vi "oopAPI_TX (SAP)_2.vi"() -> ()   [LabVIEW 2020]
uses:
  src/_polimorphicInstances/control/Fdx Start (Tx).vi
  src/AIM664LV.lvlib
  src/_polimorphicInstances/session/Fdx Close Session (Port).vi
  src/_polimorphicInstances/session/Fdx Create Session (Tx-UDP Port-Oriented).vi
  src/helpers/EthFrameManagement/EthFrameManagement.lvlib
  src/bsp/AFDX_Transmit/Fdx Create Tx VL.vi
  src/_polimorphicInstances/udpPort/Fdx Create UDP Port (TX-SAP).vi
  src/_polimorphicInstances/control/Fdx Stop (Tx).vi
  src/_controls/comm_config_vl_tx.ctl
  src/_controls/sap_config_tx.ctl
  src/_controls/comm_computedMAC-IP.ctl
panel:
  out "Duplicated":bool
  out "Array":T1[](array[typedef]) {"MACsrc" format="%.0x"}
  in  "SapPort Config":T2[](array[typedef])=[{"partitionID"=1, "SubVlId"=1, "UdpSrcPort"=1, "UdpNumBufMessages"=0, "UdpMaxMessageSize"=1000}]
  in  "VL Config":T3={"VlId"=60, "NumOfSubVl"=1, "rate mS (128)"=128.0, "domainID"=1, "sideID"=1, "locationID"=1, "interfaceID"=1, "NetSelect"=3, "Skew"=0, "MaxFrameLength"=1000, "FrameBufferSize"=0} {"NetSelect" items=["FDX_TX_FRAME_DLY_A"=0, "FDX_TX_FRAME_DLY_B"=1, "FDX_TX_FRAME_BOTH "=3, "FDX_TX_FRAME_ONLY_A"=4, "FDX_TX_FRAME_ONLY_B "=5]; "interfaceID" format="%.0b"}
  in  "VLid Dest":u32=50
  in  "UdpDst":u32=12347
  in  "Update period mS":u32=10
  in  "PortMap":u32
  out "IndexCycleCount":u32[](array[numeric])
  out "MsgCount":u32[](array[numeric])
  out "CurrentIndex":u32[](array[numeric])
  out "BytesWritten":u32[](array[numeric])
  in  "port":u32
  in  "board":u32
  out "current time":timestamp=timestamp(3677762637.591913 s since 1904-01-01)
  out "current irig time":T4={"SignOut"=40, "DayOut"=1, "HourOut"=1, "MinOut"=28, "SecondOut"=39, "MilliSecOut"=539, "MicroSecOut"=300, "NanoSecOut"=0, "InfoOut"=0, "Mode"=3}
  in  "Data":u8[](array[numeric])=[10] format="%.0x"
  in  "stop":bool
  out "PortInitOut":T5={"PortConfig"=0, "PortUsed"=1, "GlobalMemFree"=0, "SharedMemFree"=0} {"PortConfig" items=["FDX_SINGLE", "FDX_REDUNDANT"]}
  out "error out":errorcluster
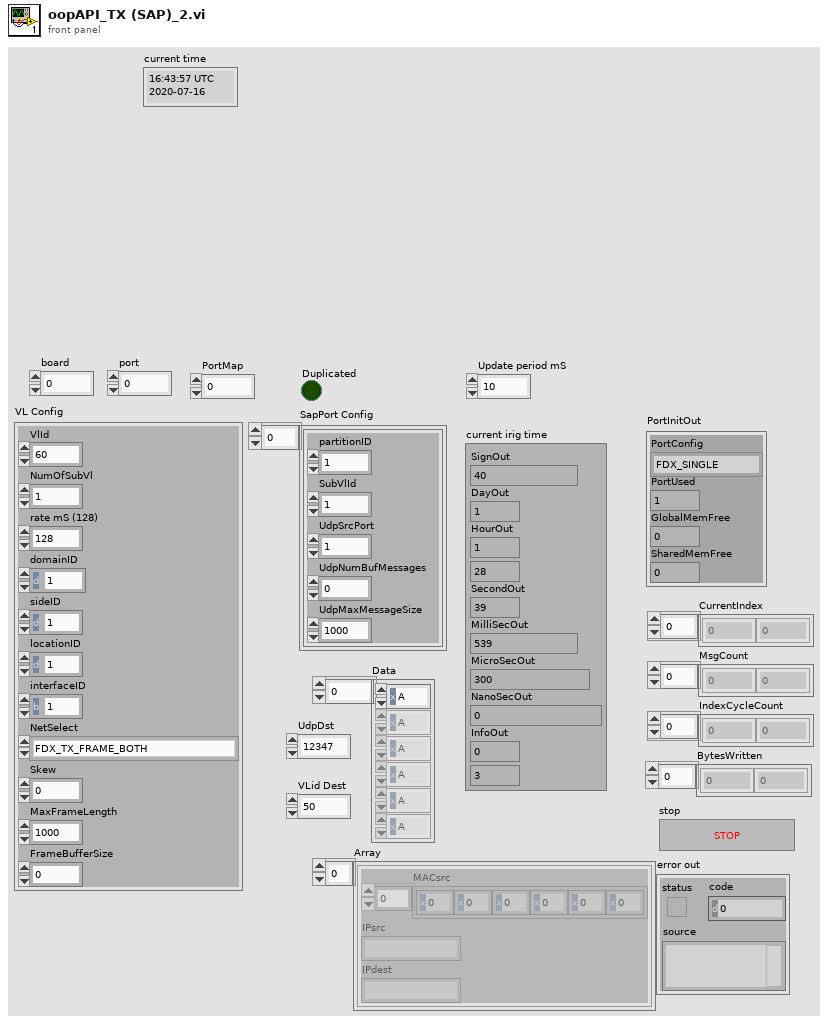
[diagram p1: front panel]
types:
  T1 = typedef "AIM664LV.lvlib/comm_computedMAC-IP.ctl" = cluster{"MACsrc":u8[], "IPsrc":string, "IPdest":string}
  T2 = typedef "AIM664LV.lvlib/sap_config_tx.ctl" = cluster{"partitionID":u8, "SubVlId":u8, "UdpSrcPort":u16, "UdpNumBufMessages":u32, "UdpMaxMessageSize":u32}
  T3 = typedef "AIM664LV.lvlib/comm_config_vl_tx.ctl" = cluster{"VlId":u16, "NumOfSubVl":u16, "rate mS (128)":dbl, "domainID":u8, "sideID":u8, "locationID":u8, "interfaceID":u8, "NetSelect":u32, "Skew":u32, "MaxFrameLength":u32, "FrameBufferSize":u32}
  T4 = cluster{"SignOut":i32, "DayOut":u32, "HourOut":u32, "MinOut":u32, "SecondOut":u32, "MilliSecOut":u32, "MicroSecOut":u32, "NanoSecOut":u32, "InfoOut":u32, "Mode":u32}
  T5 = cluster{"PortConfig":u32, "PortUsed":u32, "GlobalMemFree":u32, "SharedMemFree":u32}
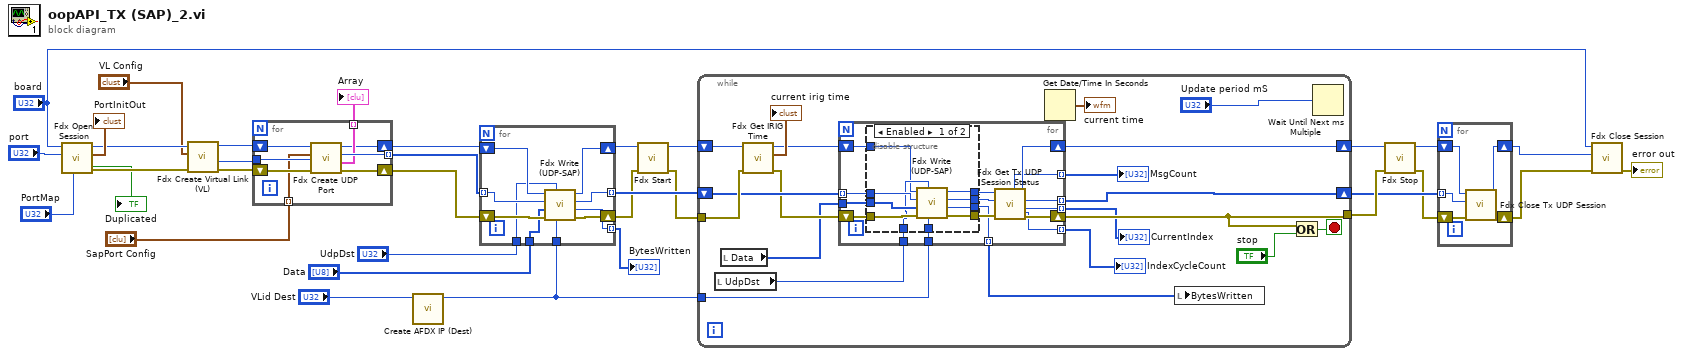
[diagram p0: block diagram]
diagram:
  n1 = call-poly "Fdx Open Session.vi"("PortMap"="PortMap", "port"="port", "board"="board") -> ("error out"=w13:errorcluster, "PortInitOut"=→"PortInitOut":T5, "port handle out"=w14:u32, "Duplicated"=→"Duplicated":bool)  [unwired: 4 in, 1 out]
  n2 = call-poly "Fdx Create Virtual Link (VL).vi"("error in (no error)"=w13, "VL Config"="VL Config", "InstrumentHandle in"=w14) -> ("error out"=w10:errorcluster, "VlId"=w9:u16, "InstrumentHandle out"=w11:u32)  [unwired: 6 in]
  n3 = for {
    tunnel: [w41] -> w32 mode=indexing
    tunnel: [w38] -> w7 mode=indexing
    shift-right: [w37] -> w5
    shift-left: w11 -> [w42]
    shift-right: [w40] -> w30
    shift-left: w10 -> [w39]
    tunnel: w9 -> [w36]
    tunnel: "SapPort Config" -> [w35] mode=indexing
    n4 = call-poly "Fdx Create UDP Port.vi"("error in (no error)"=w39, "VlId"=w36, "SapPort Config"=w35, "port handle in"=w42) -> ("error out"=w40:errorcluster, "computedAddresses"=w38:T1, "sapPort handle out"=w41:u32, "port handle out"=w37:u32)  [unwired: 4 in]
  }
  "Array" <- w7
  n5 = call "Create AFDX IP (Dest).vi"("VL"="VLid Dest") -> ("ip net"=w15:u32)  [unwired: 9 in, 1 out]
  n6 = for {
    tunnel: "Data" -> [w43]
    tunnel: [w50] -> w19 mode=indexing
    shift-right: [w51] -> w27
    shift-left: w30 -> [w52]
    tunnel: w32 -> [w45] mode=indexing
    tunnel: [w46] -> w31 mode=indexing
    tunnel: "UdpDst" -> [w44]
    tunnel: w15 -> [w49]
    shift-right: [w47] -> w4
    shift-left: w5 -> [w48]
    n7 = call "Fdx Write (UDP-SAP).vi"("IpDst"=w49, "UdpDst"=w44, "error in (no error)"=w52, "Data"=w43, "UdpHandle in"=w45, "InstrumentHandle_port in"=w48) -> ("error out"=w51:errorcluster, "BytesWritten"=w50:u32, "UdpHandle out"=w46:u32, "InstrumentHandle_port out"=w47:u32)  [unwired: 2 in]
  }
  "BytesWritten" <- w19
  n8 = call-poly "Fdx Start.vi"("error in (no error)"=w27, "InstrumentHandle_port in"=w4) -> ("error out"=w26:errorcluster, "InstrumentHandle_port out"=w25:u32)  [unwired: 8 in]
  n9 = while {
    tunnel: w26 -> [w68]
    tunnel: [w65] -> w23
    tunnel: w15 -> [w58]
    shift-right: [w55] -> w28
    shift-left: w25 -> [w69]
    shift-right: [w54] -> w22
    shift-left: w31 -> [w62]
    stop <- w71 stop-if-true
    n10 = local read "UdpDst"() -> (w57:u32)
    n11 = local read "Data"() -> (w59:u8[])
    n12 = call "Fdx Get IRIG Time.vi"("error in (no error)"=w68, "InstrumentHandle_board in"=w69) -> ("error out"=w61:errorcluster, "Curent Irig Time"=→"current irig time":T4, "InstrumentHandle_board out"=w56:u32)  [unwired: 7 in]
    n13 = for {
      tunnel: [w87] -> w64 mode=indexing
      tunnel: [w86] -> w54 mode=indexing
      tunnel: [w85] -> w63 mode=indexing
      tunnel: w62 -> [w84] mode=indexing
      tunnel: [w80] -> w60 mode=indexing
      tunnel: w59 -> [w79]
      shift-right: [w88] -> w65
      shift-left: w61 -> [w83]
      tunnel: w58 -> [w78]
      tunnel: w57 -> [w77]
      shift-right: [w74] -> w55
      shift-left: w56 -> [w76]
      tunnel: [w73] -> w53 mode=indexing
      n14 = disable-structure shown="Enabled" {
        disable-tunnel: w84 -> [w94 w100]
        disable-tunnel: w83 -> [w98 w99]
        disable-tunnel: [w97 w99] -> w82
        disable-tunnel: [w89 w100] -> w81
        disable-tunnel: [w96 _] -> w80
        disable-tunnel: w79 -> [w93 _]
        disable-tunnel: w78 -> [w95 _]
        disable-tunnel: w77 -> [w92 _]
        disable-tunnel: w76 -> [w91 _]
        disable-tunnel: [w90 _] -> w75
        frame Enabled {
          n15 = call "Fdx Write (UDP-SAP).vi"("IpDst"=w95, "UdpDst"=w92, "error in (no error)"=w98, "Data"=w93, "UdpHandle in"=w94, "InstrumentHandle_port in"=w91) -> ("error out"=w97:errorcluster, "BytesWritten"=w96:u32, "UdpHandle out"=w90:u32, "InstrumentHandle_port out"=w89:u32)  [unwired: 2 in]
        }
        frame Disabled {
        }
      }
      n16 = call "Fdx Get Tx UDP Session Status.vi"("error in (no error)"=w82, "UdpHandle in"=w75, "InstrumentHandle_port in"=w81) -> ("error out"=w88:errorcluster, "CurrentIndex"=w87:u32, "UdpHandle out"=w86:u32, "InstrumentHandle_port out"=w74:u32, "IndexCycleCount"=w85:u32, "MsgCount"=w73:u32)  [unwired: 3 in]
    }
    "CurrentIndex" <- w64
    "MsgCount" <- w53
    "IndexCycleCount" <- w63
    n17 = Get Date/Time In Seconds() -> (seconds since 1Jan1904=→"current time":timestamp)
    n18 = local write "BytesWritten"(w60) -> ()
    n19 = Or(x=w65, y="stop") -> (x .or. y?=w71:bool)
    n20 = Wait Until Next ms Multiple(millisecond multiple="Update period mS") -> ()  [unwired: 1 out]
  }
  n21 = call-poly "Fdx Stop.vi"("error in (no error)"=w23, "InstrumentHandle_port in"=w28) -> ("error out"=w21:errorcluster, "InstrumentHandle_port out"=w3:u32)  [unwired: 8 in]
  n22 = for {
    tunnel: w22 -> [w101] mode=indexing
    shift-right: [w104] -> w20
    shift-left: w21 -> [w105]
    shift-right: [w102] -> w2
    shift-left: w3 -> [w103]
    n23 = call "Fdx Close Tx UDP Session.vi"("error in (no error)"=w105, "UdpHandle in"=w101, "InstrumentHandle_port in"=w103) -> ("error out"=w104:errorcluster, "InstrumentHandle_port out"=w102:u32)  [unwired: 7 in]
  }
  n24 = call-poly "Fdx Close Session.vi"("error in (no error)"=w20, "InstrumentHandle_port in"=w2, "InstrumentHandle_board in"="board") -> ("error out"=→"error out":errorcluster)  [unwired: 8 in]
